vi "SubSystems.vi"(8 "error in":errorcluster) -> ()   [LabVIEW 2023]
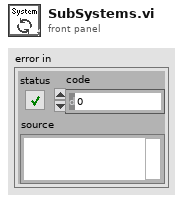
[diagram p1: front panel]
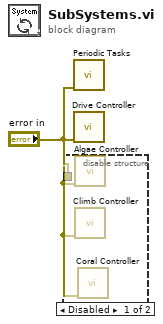
[diagram p0: block diagram]
diagram:
  n1 = disable-structure shown="Disabled" {
    disable-tunnel: "error in" -> [w2 _]
    frame Disabled {
      n2 = call "Algae Controller.vi"("error in"=w2) -> ()  [unwired: 11 in]
      n3 = call "Climb Controller.vi"("error in"=w2) -> ()  [unwired: 11 in]
      n4 = call "Coral Controller.vi"("error in"=w2) -> ()  [unwired: 10 in]
    }
    frame Enabled {
    }
  }
  n5 = call "Periodic Tasks.vi"("error in"="error in") -> ()  [unwired: 1 in, 10 out]
  n6 = call "Drive Controller.vi"("error in"="error in") -> ()  [unwired: 11 in]
